vi "Included_Point.vi"(0 "Y Centre(mm)":dbl, 2 "X Centre(mm)":dbl, 3 "Location":cluster{"x":dbl, "y":dbl, "z":dbl}, 6 "Output rectangle":T1={"X min"=-900.0, "Xmax"=900.0, "Ymin"=-1500.0, "Y max"=1500.0}) -> (1 "Included?":bool)   [LabVIEW 2010]
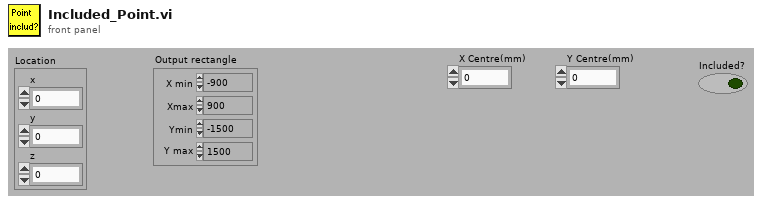
[diagram p1: front panel]
types:
  T1 = cluster{"X min":dbl, "Xmax":dbl, "Ymin":dbl, "Y max":dbl}
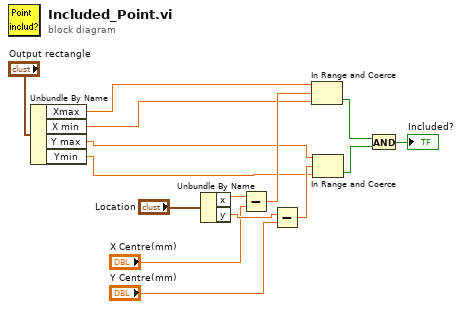
[diagram p0: block diagram]
diagram:
  n1 = Unbundle By Name("Output rectangle") -> ("Xmax"=w4:dbl, "X min"=w3:dbl, "Y max"=w2:dbl, "Ymin"=w1:dbl)
  n2 = Unbundle By Name("Location") -> ("x"=w10:dbl, "y"=w12:dbl)
  n3 = Subtract(x=w10, y="X Centre(mm)") -> (x-y=w14:dbl)
  n4 = Subtract(x=w12, y="Y Centre(mm)") -> (x-y=w15:dbl)
  n5 = In Range and Coerce(upper limit=w4, x=w14, lower limit=w3) -> (In Range?=w8:bool)  [unwired: 1 out]
  n6 = In Range and Coerce(upper limit=w2, x=w15, lower limit=w1) -> (In Range?=w7:bool)  [unwired: 1 out]
  n7 = And(x=w8, y=w7) -> (x .and. y?=→"Included?":bool)
